vi "Send_RC_Switch.vi"() -> ()   [LabVIEW 2016]
uses:
  <vilib>/DAQmx/write.llb/DAQmx Write (Digital Bool 1Line 1Point).vi
  <vilib>/DAQmx/create/channels.llb/DAQmx Create Channel (DO-Digital Output).vi
  <vilib>/DAQmx/miscellaneous.llb/DAQmx Fill In Error Info.vi
panel:
  in  "send":bool
  in  "stop":bool
  in  "error in":errorcluster
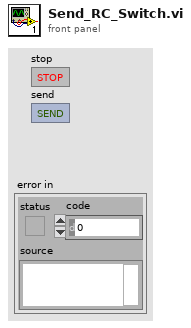
[diagram p1: front panel]
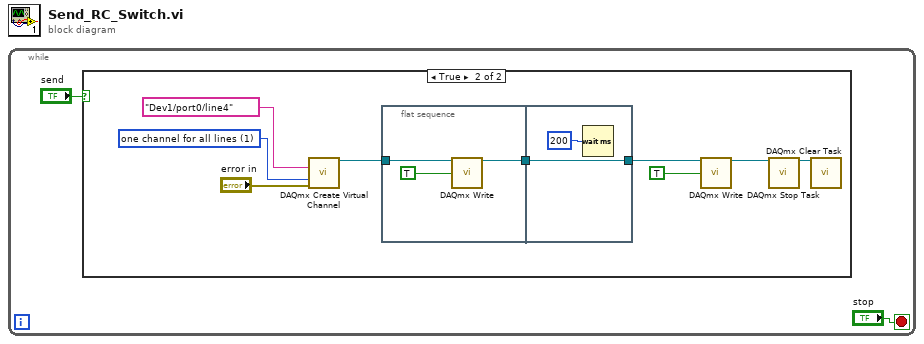
[diagram p0: block diagram]
diagram:
  n1 = while {
    stop <- "stop" stop-if-true
    n2 = case shown="True" "send" {
      frame False {
      }
      frame True {
        w9 = 1 items=["one channel for each line", "one channel for all lines"] ("line grouping")
        n3 = call-poly <vilib>:"DAQmx Create Virtual Channel.vi"("lines"=tag "Dev1/port0/line4", "line grouping"=w9, "error in"="error in") -> ("task out"=w3:refnum<k21>)  [unwired: 11 in, 1 out]
        n4 = flat-sequence {
          tunnel: [w14] -> w7
          tunnel: w3 -> [w12]
          tunnel: [w16] -> w5
          tunnel: w7 -> [w16]
          frame #0 {
            n5 = call-poly <vilib>:"DAQmx Write.vi"("task/channels in"=w12, "data"=TRUE) -> ("task out"=w14:refnum<k21>)  [unwired: 11 in, 2 out]
          }
          frame #1 {
            n6 = Wait (ms)(milliseconds to wait=u32 200) -> ()  [unwired: 1 out]
          }
        }
        n7 = call-poly <vilib>:"DAQmx Write.vi"("task/channels in"=w5, "data"=TRUE) -> ("task out"=w4:refnum<k21>)  [unwired: 11 in, 2 out]
        n8 = call <vilib>:"DAQmx Stop Task.vi"("task/channels in"=w4) -> ("task out"=w8:refnum<k21>)  [unwired: 13 in, 1 out]
        n9 = call <vilib>:"DAQmx Clear Task.vi"("task in"=w8) -> ()  [unwired: 14 in, 1 out]
      }
    }
  }
